vi "Read.vi"(8 "Error In":errorcluster, 10 "Path":path, 11 "Default Cluster":variant) -> (0 "Error Out":errorcluster, 3 "Cluster":variant)   [LabVIEW 2016, in "Configit.lvlib"]
doc: "Reads a named cluster that was written to file using Configit Write back into memory. You must call variant to data to convert the data back into the cluster format."
uses:
  Configit.lvlib
  Insert Error.vi
  GetTypeInfo.vi
  <vilib>/Waveform/DWDTOps.llb/DWDT Empty Digital.vi
  <vilib>/Waveform/DTblOps.llb/DTbl Empty Digital.vi
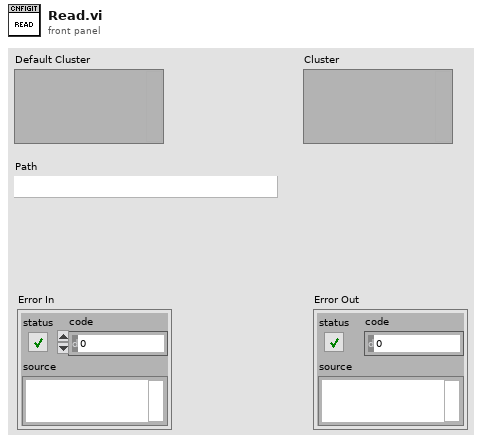
[diagram p1: front panel]
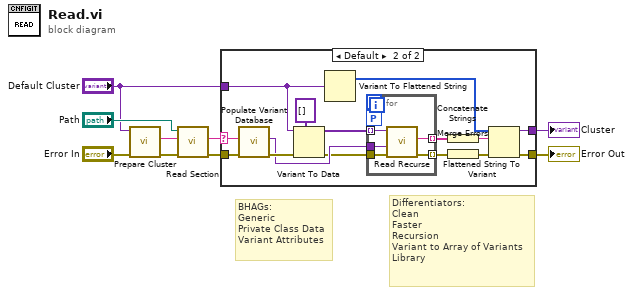
[diagram p0: block diagram]
diagram:
  # "Differentiators:\nClean\nFaster\nRecursion\nVariant to Array of Variants\nLibrary"
  # "BHAGs:\nGeneric\nPrivate Class Data\nVariant Attributes"
  n1 = call "Prepare Cluster.vi"("Error In"="Error In", "Default Cluster"="Default Cluster") -> ("Error Out"=w8:errorcluster, "Name"=w3:string)  [unwired: 8 in]
  n2 = call "Read Section.vi"("Error In"=w8, "Section"=w3, "Path"="Path") -> ("Error Out"=w6:errorcluster, "Data"=w1:string)  [unwired: 7 in]
  n3 = case shown="Default" w1 {
    selector: w1 -> [_ w12]
    tunnel: w6 -> [w10 w26]
    tunnel: [w11 w24] -> w5
    tunnel: [w10 w23] -> w4
    tunnel: "Default Cluster" -> [w11 w21]
    frame "" {
    }
    frame Default {
      n4 = call "Populate Variant Database.vi"("Error In"=w26, "Data"=w12) -> ("Error Out"=w22:errorcluster, "Variant DB"=w19:variant)  [unwired: 8 in]
      n5 = Variant To Data(error in=w22, type=variant[] [], Variant=w21) -> (data=w18:variant[], error out=w16:errorcluster)
      n6 = Variant To Flattened String(Variant=w21) -> (1:w25:i16[])  [unwired: 1 out]
      n7 = for {
        tunnel: w19 -> [w29]
        tunnel: w18 -> [w31] mode=indexing
        tunnel: [w30] -> w17 mode=indexing
        workers-P: _ -> [_]
        tunnel: w16 -> [w28]
        tunnel: [w27] -> w14 mode=indexing
        n8 = call "Read Recurse.vi"("Error In"=w28, "Variant DB"=w29, "Variant"=w31) -> ("Error Out"=w27:errorcluster, "String"=w30:string)  [unwired: 7 in]
      }
      n9 = Concatenate Strings(w17) -> (w13:string)
      n10 = Merge Errors(w14) -> (w15:errorcluster)
      n11 = Flattened String To Variant(4:w15, 6:w13, 7:w25) -> (0:w23:errorcluster, 3:w24:variant)
    }
  }
  "Error Out" <- w4
  "Cluster" <- w5
